vi "Set Strings from Ref.vi"(8 "error in (no error)":errorcluster, 9 "Language Index (0)":i32, 10 "GObj Refnum":refnum<vi>, 11 "WaveformGraph in":refnum<class "IntensityChart.lvclass">) -> (0 "error out":errorcluster, 3 "WaveformGraph out":refnum<class "IntensityChart.lvclass">)   [LabVIEW 2013, in "SET Project Data.lvlib" / "IntensityChart.lvclass"]
uses:
  IntensityChart.lvclass
  GraphChart/GraphChart.lvclass
  GObject/GObject.lvclass
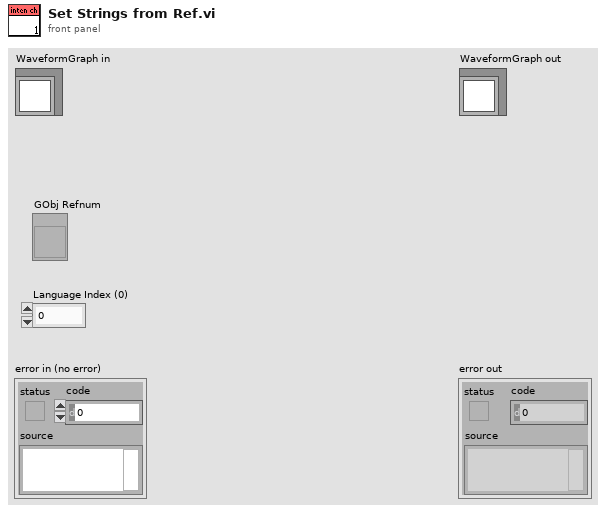
[diagram p1: front panel]
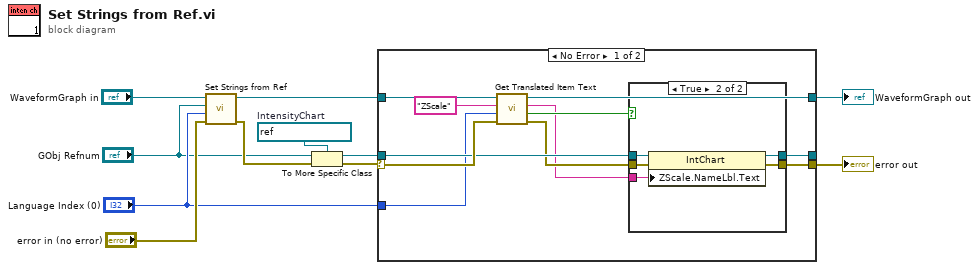
[diagram p0: block diagram]
diagram:
  w7 = refnum<vi> refnum  # IntensityChart
  n1 = call-parent "Set Strings from Ref.vi"("error in (no error)"="error in (no error)", "Language Index (0)"="Language Index (0)", "GObj Refnum"="GObj Refnum", "GraphChart in"="WaveformGraph in") -> ("error out"=w5:errorcluster, "GraphChart out"=w6:refnum<class "IntensityChart.lvclass">)  [unwired: 6 in]
  n2 = To More Specific Class(target class=w7, reference="GObj Refnum", error in=w5) -> (specific class reference=w9:refnum<vi>, error out=w8:errorcluster)
  n3 = case shown="No Error" w8 {
    selector: w8 -> [w20 w31]
    tunnel: w9 -> [w18 w30]
    tunnel: w6 -> [w21 w32]
    tunnel: "Language Index (0)" -> [w16 _]
    tunnel: [w14 w32] -> w2
    tunnel: [w12 w31] -> w1
    tunnel: [w13 w30] -> _
    frame No Error {
      n4 = call "Get Translated Item Text.vi"("error in (no error)"=w20, "LangIndex (0)"=w16, "ItemName"="ZScale", "GObject in"=w21) -> ("error out"=w17:errorcluster, "Found?"=w19:bool, "Translated Text (ASCII)"=w15:string, "GObject out"=w14:refnum<class "IntensityChart.lvclass">)  [unwired: 4 in]
      n5 = case shown="True" w19 {
        tunnel: w18 -> [w23 w29]
        tunnel: w15 -> [_ w26]
        tunnel: w17 -> [w24 w27]
        tunnel: [w24 w25] -> w12
        tunnel: [w23 w28] -> w13
        frame False {
        }
        frame True {
          n6 = property class="IntChart"(reference=w29, error in=w27, "ZScale.NameLbl.Text"=w26) -> (reference out=w28:refnum<vi>, error out=w25:errorcluster)
        }
      }
    }
    frame Error {
    }
  }
  "error out" <- w1
  "WaveformGraph out" <- w2
